vi "lettura_dati.vi"(8 "error in (no error)":errorcluster, 9 "Source Measure Unit Channel (0: Channel A)":i32(ring) items=["Channel A", "Channel B"], 10 "End Index (1)":i32=1, 11 "VISA resource name":refnum<visa-resource-name>) -> (0 "error out":errorcluster, 2 "CORRENTE":dbl[](array[numeric]), 3 "VISA resource name out":refnum<visa-resource-name>, 5 "TENSIONE":dbl[](array[numeric]), 7 "TEMPI":dbl[](array[numeric]))   [LabVIEW 2025]
uses:
  <instrlib>/Keithley 2600 Series/Keithley 2600 Series.lvlib
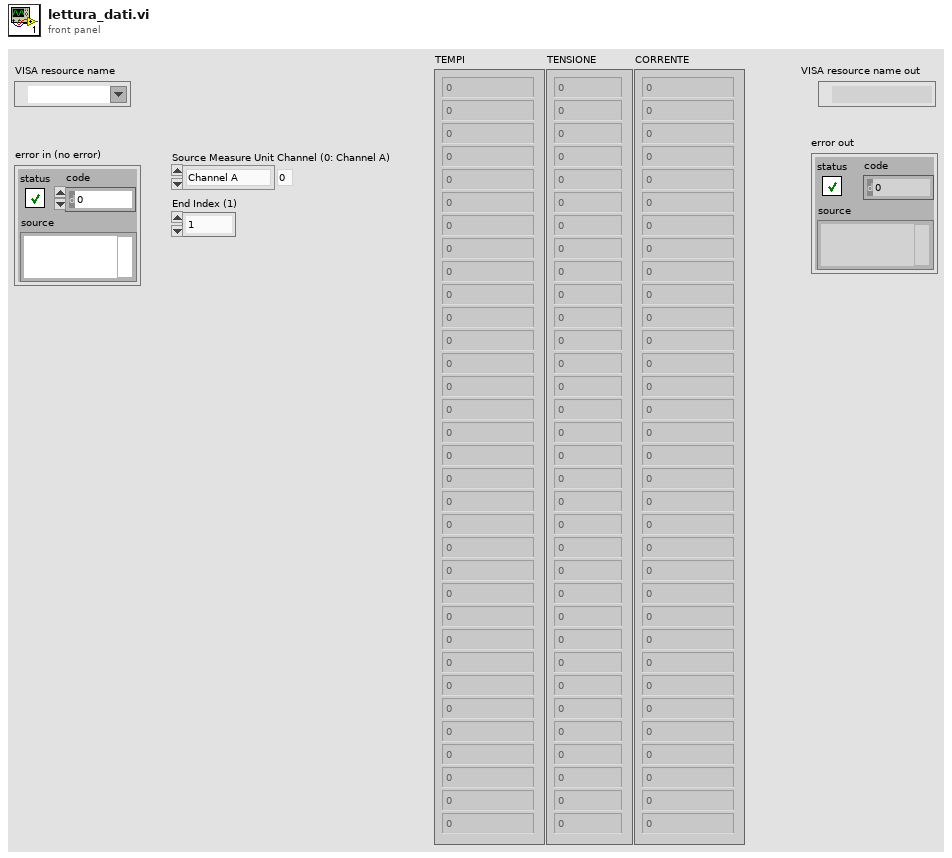
[diagram p1: front panel]
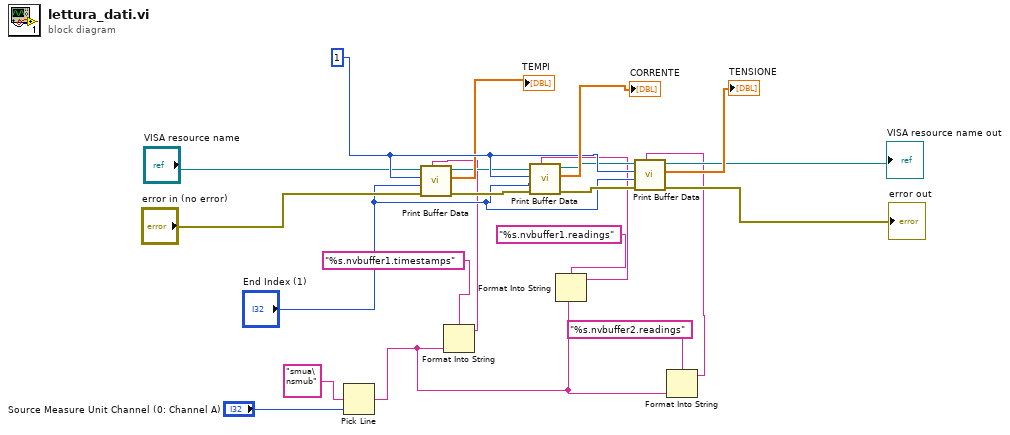
[diagram p0: block diagram]
diagram:
  w19 = 1 ("Start Index (1)")
  n1 = Pick Line(multi-line string="smua\nsmub", line index="Source Measure Unit Channel (0: Channel A)") -> (output string=w1:string)  [unwired: 1 in]
  n2 = Format Into String(format string="%s.nvbuffer1.timestamps" ("Reading Buffer (smua.nvbuffer1)"), w1) -> (resulting string=w6:string)  [unwired: 2 in, 1 out]
  n3 = call <instrlib>:"Print Buffer Data.vi"("Reading Buffer (smua.nvbuffer1)"=w6, "error in (no error)"="error in (no error)", "End Index (1)"="End Index (1)", "Start Index (1)"=w19, "VISA resource name"="VISA resource name") -> ("Buffer Data"=→"TEMPI":dbl[], "VISA resource name out"=w14:refnum<visa-resource-name>)  [unwired: 4 in, 1 out]
  n4 = Format Into String(format string="%s.nvbuffer1.readings" ("Reading Buffer (smua.nvbuffer1)"), w1) -> (resulting string=w5:string)  [unwired: 2 in, 1 out]
  n5 = call <instrlib>:"Print Buffer Data.vi"("Reading Buffer (smua.nvbuffer1)"=w5, "error in (no error)"="error in (no error)", "End Index (1)"="End Index (1)", "Start Index (1)"=w19, "VISA resource name"=w14) -> ("error out"=w17:errorcluster, "Buffer Data"=→"CORRENTE":dbl[], "VISA resource name out"=w13:refnum<visa-resource-name>)  [unwired: 4 in]
  n6 = Format Into String(format string="%s.nvbuffer2.readings" ("Reading Buffer (smua.nvbuffer1)"), w1) -> (resulting string=w3:string)  [unwired: 2 in, 1 out]
  n7 = call <instrlib>:"Print Buffer Data.vi"("Reading Buffer (smua.nvbuffer1)"=w3, "error in (no error)"=w17, "End Index (1)"="End Index (1)", "Start Index (1)"=w19, "VISA resource name"=w13) -> ("error out"=→"error out":errorcluster, "Buffer Data"=→"TENSIONE":dbl[], "VISA resource name out"=→"VISA resource name out":refnum<visa-resource-name>)  [unwired: 4 in]
